vi "Write Status.vi"(8 "error in":errorcluster, 10 "Status in":string, 11 "File IO.lvclass in":refnum<class "File IO.lvclass">) -> (0 "error out":errorcluster, 3 "File IO.lvclass out":refnum<class "File IO.lvclass">)   [LabVIEW 2017, in "File IO.lvclass"]
uses:
  File IO.lvclass
  File IO.lvclass/File IO.ctl
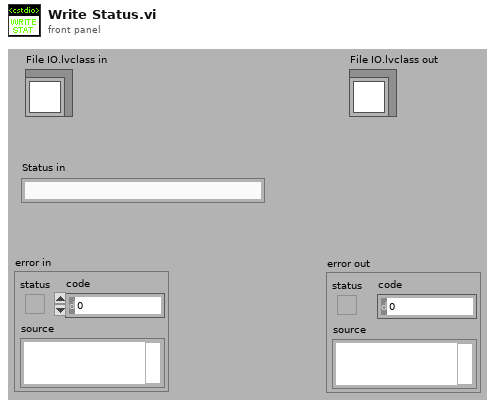
[diagram p1: front panel]
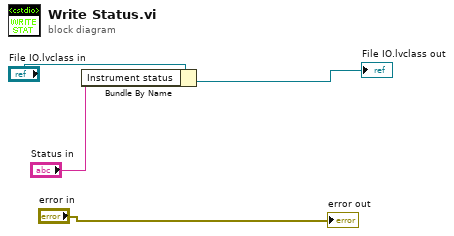
[diagram p0: block diagram]
diagram:
  n1 = Bundle By Name(cluster="File IO.lvclass in", "Instrument status"="Status in") -> (→"File IO.lvclass out":refnum<class "File IO.lvclass">)
  "error out" <- "error in"
